vi "Function_request_status.vi"(5 "VISA resource name in":refnum<visa-resource-name>, 7 "error in":errorcluster, 10 "Direction":string, 11 "Server addr":string) -> (3 "Dispensed1":string, 4 "VISA resource name out":refnum<visa-resource-name>, 6 "error out":errorcluster)   [LabVIEW 2020]
panel:
  out "return count":u32
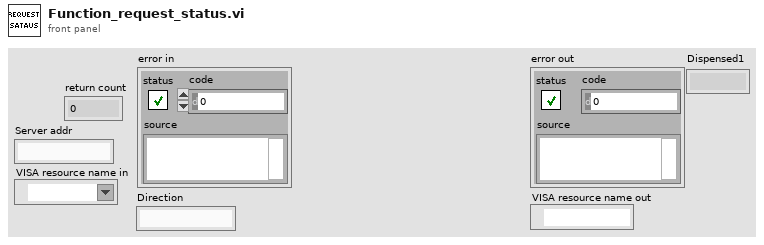
[diagram p1: front panel]
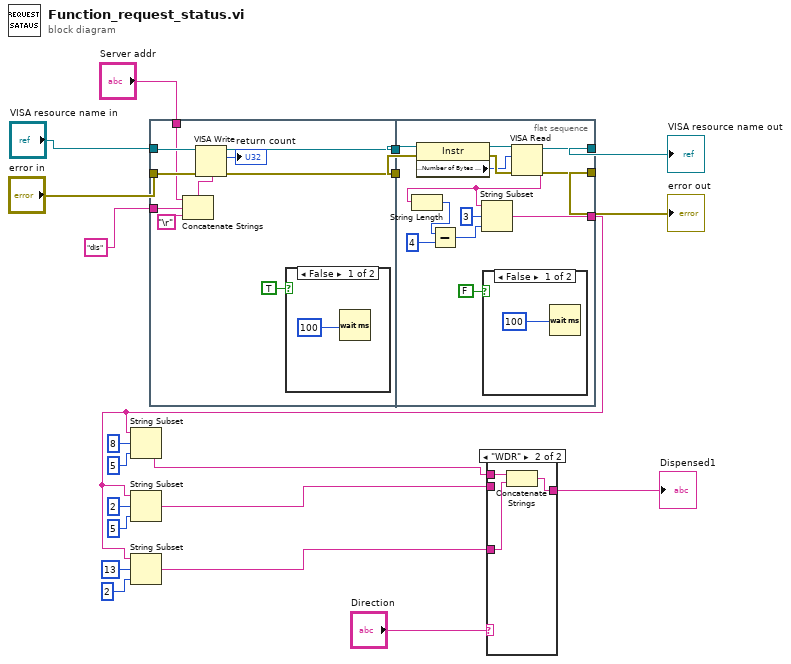
[diagram p0: block diagram]
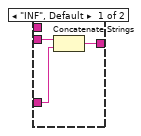
[diagram p4: hidden frame]
diagram:
  n1 = String Subset(string=w6, offset (0)=8, length (rest)=5 ("length (rest)")) -> (substring=w10:string)
  n2 = String Subset(string=w6, offset (0)=2, length (rest)=5 ("length (rest)")) -> (substring=w11:string)
  n3 = String Subset(string=w6, offset (0)=13, length (rest)=2 ("length (rest)")) -> (substring=w12:string)
  n4 = flat-sequence {
    tunnel: "VISA resource name in" -> [w30]
    tunnel: "error in" -> [w29]
    tunnel: "Server addr" -> [w28]
    tunnel: "dis" ("string") -> [w27]
    tunnel: [w25] -> w20
    tunnel: [w24] -> w19
    tunnel: w20 -> [w45]
    tunnel: w19 -> [w44]
    tunnel: [w40] -> w7
    tunnel: [w39] -> w5
    tunnel: [w33] -> w6
    frame #0 {
      n5 = Concatenate Strings(w28, w27, "\r") -> (w26:string)
      n6 = VISA Write(VISA resource name=w30, write buffer=w26, error in (no error)=w29) -> (VISA resource name out=w25:refnum<visa-resource-name>, return count=→"return count":u32, error out=w24:errorcluster)
      n7 = case shown="False" TRUE {
        frame False {
          n8 = Wait (ms)(milliseconds to wait=u32 100) -> ()  [unwired: 1 out]
        }
        frame True {
        }
      }
    }
    frame #1 {
      n9 = property class="Instr"(reference=w45, error in=w44) -> (reference out=w43:refnum<visa-resource-name>, error out=w42:errorcluster, "Serial Settings:Number of Bytes at Serial Port"=w41:u32)
      n10 = case shown="False" FALSE {
        frame False {
          n11 = Wait (ms)(milliseconds to wait=u32 100) -> ()  [unwired: 1 out]
        }
        frame True {
        }
      }
      n12 = VISA Read(VISA resource name=w43, byte count=w41, error in (no error)=w42) -> (VISA resource name out=w40:refnum<visa-resource-name>, read buffer=w34:string, error out=w39:errorcluster)  [unwired: 1 out]
      n13 = String Length(string=w34) -> (length=w37:i32)
      n14 = Subtract(x=w37, y=4) -> (x-y=w35:i32)
      n15 = String Subset(string=w34, offset (0)=3, length (rest)=w35) -> (substring=w33:string)
    }
  }
  n16 = case shown="\"WDR\"" "Direction" {
    tunnel: [w49 w52] -> w1
    tunnel: w12 -> [w48 w50]
    tunnel: w11 -> [w47 _]
    tunnel: w10 -> [_ w51]
    frame "INF", Default {
      n17 = Concatenate Strings(w47, w48) -> (w49:string)
    }
    frame "WDR" {
      n18 = Concatenate Strings(w51, w50) -> (w52:string)
    }
  }
  "Dispensed1" <- w1
  "error out" <- w5
  "VISA resource name out" <- w7
